vi "Leap Motion Controller Help.vi"   [LabVIEW 2010]
uses:
  <vilib>/Platform/browser.llb/Open URL in Default Browser (string).vi
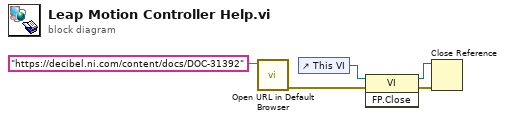
[diagram p0: block diagram]
diagram:
  n1 = call-poly <vilib>:"Open URL in Default Browser.vi"("URL"="https://decibel.ni.com/content/docs/DOC-31392") -> ("error out"=w2:errorcluster)  [unwired: 5 in, 1 out]
  n2 = control-ref of="This VI"() -> (w5:refnum<vi>)
  n3 = invoke class="VI" method="FP.Close"(reference=w5, error in=w2) -> (reference out=w3:refnum<vi>, error out=w4:errorcluster)  [unwired: 1 in, 1 out]
  n4 = Close Reference(reference=w3, error in (no error)=w4) -> ()  [unwired: 1 out]
